vi "Focus Stop.vi"(8 "error in (no error)":errorcluster, 10 "Motor (0:n-1)":i32, 11 "NewFocus in":refnum<class "NewFocus.lvclass">) -> (0 "error out":errorcluster, 3 "NewFocus out":refnum<class "NewFocus.lvclass">)   [LabVIEW 2024, in "NewFocus.lvclass"]
uses:
  NewFocus.lvclass
  NewFocus.lvclass/NewFocus.ctl
  Focus Class/Focus Class.lvclass
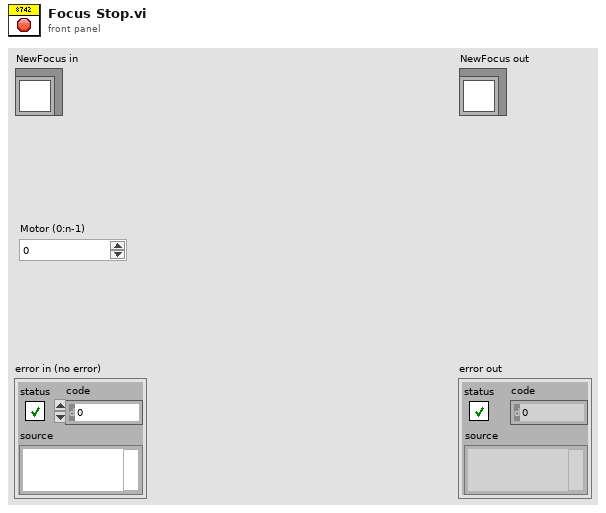
[diagram p1: front panel]
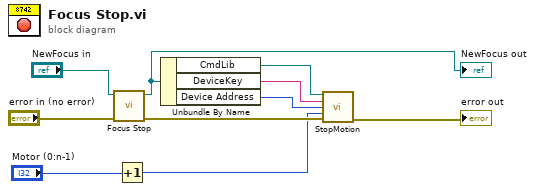
[diagram p0: block diagram]
diagram:
  n1 = call-parent "Focus Stop.vi"("error in (no error)"="error in (no error)", "Focus Class in"="NewFocus in") -> ("error out"=w5:errorcluster, "Focus Class out"=w3:refnum<class "NewFocus.lvclass">)  [unwired: 8 in]
  "NewFocus out" <- w3
  n2 = Increment(x="Motor (0:n-1)") -> (x+1=w1:i32)
  n3 = Unbundle By Name(w3) -> ("CmdLib"=w8:refnum<k24>, "DeviceKey"=w7:string, "Device Address"=w6:i32)
  n4 = call "StopMotion.vi"("CmdLib In"=w8, "DeviceKey In"=w7, "Device Address In"=w6, "Motor"=w1, "error in (no error)"=w5) -> ("error out"=→"error out":errorcluster)  [unwired: 7 in, 3 out]
